vi "Lab Panel V5.25.1.vi"() -> ()   [LabVIEW 2013] (continued)
                            n2538 = local write "data file error"(w4596) -> ()
                          }
                        }
                      }
                    }
                  }
                }
              }
              frame #8 {
                n2539 = case shown="True" w4635 {
                  tunnel: w4639 -> [_ w4644]
                  tunnel: w4638 -> [_ w4643]
                  tunnel: w4637 -> [_ w4641]
                  tunnel: w4636 -> [_ w4640]
                  frame False {
                  }
                  frame True {
                    n2540 = local read "DISP LAB05-1"() -> (w4645:T4)
                    n2541 = local read "SIG LAB05-1"() -> (w4646:T2)
                    n2542 = local read "ON L05-1"() -> (w4642:cluster{"amps":dbl, "volts":dbl, "pf":dbl})
                    n2543 = Unbundle(w4646) -> ("AMPS"=w4652:dbl, "VOLTS"=w4650:dbl, "PF"=w4649:dbl, "Tmp Live"=w4648:dbl, "Tmp Neut"=w4651:dbl)
                    n2544 = Unbundle(w4645) -> ("CYCLE"=w4647:dbl)  [unwired: 2 out]
                    n2545 = stacked-sequence {
                      tunnel: w4652 -> [w4656 w4675]
                      tunnel: w4651 -> [_ w4674]
                      tunnel: w4650 -> [w4655 w4673]
                      tunnel: w4649 -> [w4654 w4672]
                      tunnel: w4648 -> [_ w4671]
                      tunnel: w4647 -> [_ w4670]
                      tunnel: w4644 -> [_ w4669]
                      tunnel: w4643 -> [w4657 _]
                      tunnel: w4642 -> [w4653 w4667]
                      tunnel: w4641 -> [_ w4668]
                      tunnel: w4640 -> [_ w4663]
                      frame #0 {
                        n2546 = case shown="True" w4657 {
                          tunnel: w4656 -> [_ w4662]
                          tunnel: w4655 -> [_ w4661]
                          tunnel: w4654 -> [_ w4660]
                          tunnel: w4653 -> [_ w4658]
                          frame False {
                          }
                          frame True {
                            n2547 = Bundle(cluster=w4658, "amps"=w4662, "volts"=w4661, "pf"=w4660) -> (w4659:cluster{"amps":dbl, "volts":dbl, "pf":dbl})
                            n2548 = local write "ON L05-1"(w4659) -> ()
                          }
                        }
                      }
                      frame #1 {
                        n2549 = Unbundle(w4667) -> ("amps"=w4666:dbl, "volts"=w4665:dbl, "pf"=w4664:dbl)
                        n2550 = case shown="True" w4668 {
                          tunnel: w4675 -> [_ w4707]
                          tunnel: w4674 -> [_ w4714]
                          tunnel: w4673 -> [_ _]
                          tunnel: w4672 -> [_ _]
                          tunnel: w4671 -> [_ w4713]
                          tunnel: w4670 -> [_ w4712]
                          tunnel: w4669 -> [_ w4677]
                          tunnel: w4666 -> [_ w4709]
                          tunnel: w4665 -> [_ w4708]
                          tunnel: w4664 -> [_ w4706]
                          tunnel: w4663 -> [_ w4698]
                          frame False {
                          }
                          frame True {
                            n2551 = local read "TDMS LAB05-1"() -> (w4711:refnum<k34>)
                            n2552 = Build Array(w4708) -> (w4703:dbl[])
                            n2553 = Build Array(w4706) -> (w4702:dbl[])
                            n2554 = Build Array(w4713) -> (w4701:dbl[])
                            n2555 = Build Array(w4714) -> (w4700:dbl[])
                            n2556 = Build Array(w4709) -> (w4705:dbl[])
                            n2557 = Build Array(w4707) -> (w4704:dbl[])
                            n2558 = Build Array(w4712) -> (w4699:dbl[])
                            n2559 = Build Array("AMPS ON", "AMPS OFF", "VOLTS", "PF", "TEMP Live", "TEMP Neut", "CYCLE") -> (w4682:string[])
                            n2560 = Bundle By Name("Y"=w4705, "t0"=w4698) -> (w4697:waveform(dbl))  [unwired: 1 in]
                            n2561 = Bundle By Name("Y"=w4704, "t0"=w4698) -> (w4696:waveform(dbl))  [unwired: 1 in]
                            n2562 = Bundle By Name("Y"=w4703, "t0"=w4698) -> (w4695:waveform(dbl))  [unwired: 1 in]
                            n2563 = Bundle By Name("Y"=w4702, "t0"=w4698) -> (w4694:waveform(dbl))  [unwired: 1 in]
                            n2564 = Bundle By Name("Y"=w4701, "t0"=w4698) -> (w4693:waveform(dbl))  [unwired: 1 in]
                            n2565 = Bundle By Name("Y"=w4700, "t0"=w4698) -> (w4692:waveform(dbl))  [unwired: 1 in]
                            n2566 = Bundle By Name("Y"=w4699, "t0"=w4698) -> (w4691:waveform(dbl))  [unwired: 1 in]
                            n2567 = Build Array(w4697, w4696, w4695, w4694, w4693, w4692, w4691) -> (w4690:waveform(dbl)[])
                            n2568 = TDMS Write(0:w4711, 5:"TEST VALUES", 7:w4682, 9:w4690) -> (4:w4681:refnum<k34>, 6:w4680:string, 15:w4679:errorcluster)  [unwired: 2 in, 1 out]
                            n2569 = TDMS Write(0:w4681, 5:w4680, 7:"TIME", 9:w4677, 11:w4679) -> (15:w4676:errorcluster)  [unwired: 1 in, 3 out]
                            n2570 = local write "data file error"(w4676) -> ()
                          }
                        }
                      }
                    }
                  }
                }
              }
              frame #9 {
                n2571 = case shown="True" w4715 {
                  tunnel: w4719 -> [_ w4724]
                  tunnel: w4718 -> [_ w4723]
                  tunnel: w4717 -> [_ w4721]
                  tunnel: w4716 -> [_ w4720]
                  frame False {
                  }
                  frame True {
                    n2572 = local read "DISP LAB05-2"() -> (w4725:T4)
                    n2573 = local read "SIG LAB05-2"() -> (w4726:T2)
                    n2574 = local read "ON L05-2"() -> (w4722:cluster{"amps":dbl, "volts":dbl, "pf":dbl})
                    n2575 = Unbundle(w4726) -> ("AMPS"=w4732:dbl, "VOLTS"=w4730:dbl, "PF"=w4729:dbl, "Tmp Live"=w4728:dbl, "Tmp Neut"=w4731:dbl)
                    n2576 = Unbundle(w4725) -> ("CYCLE"=w4727:dbl)  [unwired: 2 out]
                    n2577 = stacked-sequence {
                      tunnel: w4732 -> [w4736 w4755]
                      tunnel: w4731 -> [_ w4754]
                      tunnel: w4730 -> [w4735 w4753]
                      tunnel: w4729 -> [w4734 w4752]
                      tunnel: w4728 -> [_ w4751]
                      tunnel: w4727 -> [_ w4750]
                      tunnel: w4724 -> [_ w4749]
                      tunnel: w4723 -> [w4737 _]
                      tunnel: w4722 -> [w4733 w4747]
                      tunnel: w4721 -> [_ w4748]
                      tunnel: w4720 -> [_ w4743]
                      frame #0 {
                        n2578 = case shown="True" w4737 {
                          tunnel: w4736 -> [_ w4742]
                          tunnel: w4735 -> [_ w4741]
                          tunnel: w4734 -> [_ w4740]
                          tunnel: w4733 -> [_ w4738]
                          frame False {
                          }
                          frame True {
                            n2579 = Bundle(cluster=w4738, "amps"=w4742, "volts"=w4741, "pf"=w4740) -> (w4739:cluster{"amps":dbl, "volts":dbl, "pf":dbl})
                            n2580 = local write "ON L05-2"(w4739) -> ()
                          }
                        }
                      }
                      frame #1 {
                        n2581 = Unbundle(w4747) -> ("amps"=w4746:dbl, "volts"=w4745:dbl, "pf"=w4744:dbl)
                        n2582 = case shown="True" w4748 {
                          tunnel: w4755 -> [_ w4787]
                          tunnel: w4754 -> [_ w4794]
                          tunnel: w4753 -> [_ _]
                          tunnel: w4752 -> [_ _]
                          tunnel: w4751 -> [_ w4793]
                          tunnel: w4750 -> [_ w4792]
                          tunnel: w4749 -> [_ w4757]
                          tunnel: w4746 -> [_ w4789]
                          tunnel: w4745 -> [_ w4788]
                          tunnel: w4744 -> [_ w4786]
                          tunnel: w4743 -> [_ w4778]
                          frame False {
                          }
                          frame True {
                            n2583 = local read "TDMS LAB05-2"() -> (w4791:refnum<k34>)
                            n2584 = Build Array(w4788) -> (w4783:dbl[])
                            n2585 = Build Array(w4786) -> (w4782:dbl[])
                            n2586 = Build Array(w4793) -> (w4781:dbl[])
                            n2587 = Build Array(w4794) -> (w4780:dbl[])
                            n2588 = Build Array(w4789) -> (w4785:dbl[])
                            n2589 = Build Array(w4787) -> (w4784:dbl[])
                            n2590 = Build Array(w4792) -> (w4779:dbl[])
                            n2591 = Build Array("AMPS ON", "AMPS OFF", "VOLTS", "PF", "TEMP Live", "TEMP Neut", "CYCLE") -> (w4762:string[])
                            n2592 = Bundle By Name("Y"=w4785, "t0"=w4778) -> (w4777:waveform(dbl))  [unwired: 1 in]
                            n2593 = Bundle By Name("Y"=w4784, "t0"=w4778) -> (w4776:waveform(dbl))  [unwired: 1 in]
                            n2594 = Bundle By Name("Y"=w4783, "t0"=w4778) -> (w4775:waveform(dbl))  [unwired: 1 in]
                            n2595 = Bundle By Name("Y"=w4782, "t0"=w4778) -> (w4774:waveform(dbl))  [unwired: 1 in]
                            n2596 = Bundle By Name("Y"=w4781, "t0"=w4778) -> (w4773:waveform(dbl))  [unwired: 1 in]
                            n2597 = Bundle By Name("Y"=w4780, "t0"=w4778) -> (w4772:waveform(dbl))  [unwired: 1 in]
                            n2598 = Bundle By Name("Y"=w4779, "t0"=w4778) -> (w4771:waveform(dbl))  [unwired: 1 in]
                            n2599 = Build Array(w4777, w4776, w4775, w4774, w4773, w4772, w4771) -> (w4770:waveform(dbl)[])
                            n2600 = TDMS Write(0:w4791, 5:"TEST VALUES", 7:w4762, 9:w4770) -> (4:w4761:refnum<k34>, 6:w4760:string, 15:w4759:errorcluster)  [unwired: 2 in, 1 out]
                            n2601 = TDMS Write(0:w4761, 5:w4760, 7:"TIME", 9:w4757, 11:w4759) -> (15:w4756:errorcluster)  [unwired: 1 in, 3 out]
                            n2602 = local write "data file error"(w4756) -> ()
                          }
                        }
                      }
                    }
                  }
                }
              }
            }
          }
          frame #15 {
            # "display test values on chart"
            n2603 = local read "jig cycle"() -> (w4799:dbl)
            n2604 = local read "on loops"() -> (w4801:dbl)
            n2605 = Add(x=w4801, y=4) -> (x+y=w4798:dbl)
            n2606 = Equal?(x=w4799, y=3) -> (x = y?=w4797:bool)
            n2607 = Equal?(x=w4799, y=w4798) -> (x = y?=w4796:bool)
            n2608 = Or(x=w4797, y=w4796) -> (x .or. y?=w4795:bool)
            "graph flag" <- w4795
            n2609 = global write "Global display 3.vi" "graph flag"(w4795) -> ()
            n2610 = case shown="True" w4795 {
              frame False {
              }
              frame True {
                n2611 = local read "SIG LAB05-1"() -> (w4844:T2)
                n2612 = local read "SIG LAB04-2"() -> (w4845:T2)
                n2613 = local read "SIG LAB05-2"() -> (w4843:T2)
                n2614 = local read "SIG LAB04-1"() -> (w4846:T2)
                n2615 = local read "SIG LAB03-1"() -> (w4848:T2)
                n2616 = local read "SIG LAB03-2"() -> (w4847:T2)
                n2617 = local read "SIG LAB01-1"() -> (w4852:T2)
                n2618 = local read "SIG LAB02-2"() -> (w4849:T2)
                n2619 = local read "SIG LAB02-1"() -> (w4850:T2)
                n2620 = local read "SIG LAB01-2"() -> (w4851:T2)
                n2621 = Unbundle(w4845) -> ("AMPS"=w4835:dbl, "VOLTS"=w4825:dbl, "Tmp Live"=w4815:dbl, "Tmp Neut"=w4805:dbl)  [unwired: 1 out]
                n2622 = Unbundle(w4844) -> ("AMPS"=w4834:dbl, "VOLTS"=w4824:dbl, "Tmp Live"=w4814:dbl, "Tmp Neut"=w4804:dbl)  [unwired: 1 out]
                n2623 = Unbundle(w4843) -> ("AMPS"=w4833:dbl, "VOLTS"=w4823:dbl, "Tmp Live"=w4813:dbl, "Tmp Neut"=w4803:dbl)  [unwired: 1 out]
                n2624 = Unbundle(w4846) -> ("AMPS"=w4836:dbl, "VOLTS"=w4826:dbl, "Tmp Live"=w4816:dbl, "Tmp Neut"=w4806:dbl)  [unwired: 1 out]
                n2625 = Unbundle(w4847) -> ("AMPS"=w4837:dbl, "VOLTS"=w4827:dbl, "Tmp Live"=w4817:dbl, "Tmp Neut"=w4807:dbl)  [unwired: 1 out]
                n2626 = Unbundle(w4848) -> ("AMPS"=w4838:dbl, "VOLTS"=w4828:dbl, "Tmp Live"=w4818:dbl, "Tmp Neut"=w4808:dbl)  [unwired: 1 out]
                n2627 = Unbundle(w4849) -> ("AMPS"=w4839:dbl, "VOLTS"=w4829:dbl, "Tmp Live"=w4819:dbl, "Tmp Neut"=w4809:dbl)  [unwired: 1 out]
                n2628 = Unbundle(w4850) -> ("AMPS"=w4840:dbl, "VOLTS"=w4830:dbl, "Tmp Live"=w4820:dbl, "Tmp Neut"=w4810:dbl)  [unwired: 1 out]
                n2629 = Unbundle(w4852) -> ("AMPS"=w4842:dbl, "VOLTS"=w4832:dbl, "Tmp Live"=w4822:dbl, "Tmp Neut"=w4812:dbl)  [unwired: 1 out]
                n2630 = Unbundle(w4851) -> ("AMPS"=w4841:dbl, "VOLTS"=w4831:dbl, "Tmp Live"=w4821:dbl, "Tmp Neut"=w4811:dbl)  [unwired: 1 out]
                n2631 = stacked-sequence {
                  tunnel: w4842 -> [w4884 _ _]
                  tunnel: w4841 -> [w4883 _ _]
                  tunnel: w4840 -> [w4874 _ _]
                  tunnel: w4839 -> [w4873 _ _]
                  tunnel: w4838 -> [w4863 _ _]
                  tunnel: w4837 -> [w4862 _ _]
                  tunnel: w4836 -> [_ w4907 _]
                  tunnel: w4835 -> [_ w4906 _]
                  tunnel: w4834 -> [_ w4896 _]
                  tunnel: w4833 -> [_ w4895 _]
                  tunnel: w4832 -> [w4881 _ _]
                  tunnel: w4831 -> [w4880 _ _]
                  tunnel: w4830 -> [w4871 _ _]
                  tunnel: w4829 -> [w4870 _ _]
                  tunnel: w4828 -> [w4861 _ _]
                  tunnel: w4827 -> [w4860 _ _]
                  tunnel: w4826 -> [_ w4905 _]
                  tunnel: w4825 -> [_ w4904 _]
                  tunnel: w4824 -> [_ w4894 _]
                  tunnel: w4823 -> [_ w4893 _]
                  tunnel: w4822 -> [w4878 _ _]
                  tunnel: w4821 -> [w4876 _ _]
                  tunnel: w4820 -> [w4867 _ _]
                  tunnel: w4819 -> [w4865 _ _]
                  tunnel: w4818 -> [w4859 _ _]
                  tunnel: w4817 -> [w4857 _ _]
                  tunnel: w4816 -> [_ w4903 _]
                  tunnel: w4815 -> [_ w4901 _]
                  tunnel: w4814 -> [_ w4892 _]
                  tunnel: w4813 -> [_ w4890 _]
                  tunnel: w4812 -> [w4877 _ _]
                  tunnel: w4811 -> [w4875 _ _]
                  tunnel: w4810 -> [w4866 _ _]
                  tunnel: w4809 -> [w4864 _ _]
                  tunnel: w4808 -> [w4858 _ _]
                  tunnel: w4807 -> [w4856 _ _]
                  tunnel: w4806 -> [_ w4902 _]
                  tunnel: w4805 -> [_ w4900 _]
                  tunnel: w4804 -> [_ w4891 _]
                  tunnel: w4803 -> [_ w4889 _]
                  frame #0 {
                    n2632 = Merge Signals(w4884, w4883) -> (→"LAB01 AMPS":dynamicdata)
                    n2633 = Merge Signals(w4881, w4880) -> (→"LAB01 VOLTS":dynamicdata)
                    n2634 = Merge Signals(w4861, w4860) -> (→"LAB03 VOLTS":dynamicdata)
                    n2635 = Merge Signals(w4878, w4877, w4876, w4875) -> (→"LAB01 deg C":dynamicdata)
                    n2636 = Merge Signals(w4874, w4873) -> (→"LAB02 AMPS":dynamicdata)
                    n2637 = Merge Signals(w4867, w4866, w4865, w4864) -> (→"LAB02 deg C":dynamicdata)
                    n2638 = Merge Signals(w4859, w4858, w4857, w4856) -> (→"LAB03 deg C":dynamicdata)
                    n2639 = Merge Signals(w4871, w4870) -> (→"LAB02 VOLTS":dynamicdata)
                    n2640 = Merge Signals(w4863, w4862) -> (→"LAB03 AMPS":dynamicdata)
                  }
                  frame #1 {
                    n2641 = Merge Signals(w4894, w4893) -> (→"LAB05 VOLTS":dynamicdata)
                    n2642 = Merge Signals(w4907, w4906) -> (→"LAB04 AMPS":dynamicdata)
                    n2643 = Merge Signals(w4896, w4895) -> (→"LAB05 AMPS":dynamicdata)
                    n2644 = Merge Signals(w4892, w4891, w4890, w4889) -> (→"LAB05 deg C":dynamicdata)
                    n2645 = Merge Signals(w4903, w4902, w4901, w4900) -> (→"LAB04 deg C":dynamicdata)
                    n2646 = Merge Signals(w4905, w4904) -> (→"LAB04 VOLTS":dynamicdata)
                  }
                  frame #2 {
                    n2647 = local read "LAB05 VOLTS"() -> (w4915:dynamicdata)
                    n2648 = local read "LAB04 VOLTS"() -> (w4916:dynamicdata)
                    n2649 = local read "LAB02 VOLTS"() -> (w4918:dynamicdata)
                    n2650 = local read "LAB03 VOLTS"() -> (w4917:dynamicdata)
                    n2651 = local read "LAB05 AMPS"() -> (w4921:dynamicdata)
                    n2652 = local read "LAB01 VOLTS"() -> (w4919:dynamicdata)
                    n2653 = local read "LAB04 AMPS"() -> (w4922:dynamicdata)
                    n2654 = local read "LAB03 AMPS"() -> (w4923:dynamicdata)
                    n2655 = local read "LAB03 deg C"() -> (w4911:dynamicdata)
                    n2656 = local read "LAB02 AMPS"() -> (w4924:dynamicdata)
                    n2657 = local read "LAB04 deg C"() -> (w4910:dynamicdata)
                    n2658 = local read "LAB05 deg C"() -> (w4909:dynamicdata)
                    n2659 = local read "LAB02 deg C"() -> (w4912:dynamicdata)
                    n2660 = local read "LAB01 deg C"() -> (w4913:dynamicdata)
                    n2661 = local read "LAB01 AMPS"() -> (w4925:dynamicdata)
                    n2662 = Merge Signals(w4913, w4912, w4911, w4910, w4909) -> (w4908:dynamicdata)
                    n2663 = Merge Signals(w4925, w4924, w4923, w4922, w4921) -> (w4920:dynamicdata)
                    n2664 = Merge Signals(w4919, w4918, w4917, w4916, w4915) -> (w4914:dynamicdata)
                    n2665 = global write "Global display 3.vi" "graph volts"(w4914) -> ()
                    n2666 = global write "Global display 3.vi" "graph deg C"(w4908) -> ()
                    n2667 = global write "Global display 3.vi" "graph amps"(w4920) -> ()
                  }
                }
              }
            }
          }
          frame #16 {
            # "check for amps fail"
            # "check for cycle test & temperature rise fail conditions"
            n2668 = local read "on loops"() -> (w4952:dbl)
            n2669 = local read "jig cycle"() -> (w4949:dbl)
            n2670 = local read "jig cycle"() -> (w4954:dbl)
            n2671 = Add(x=w4952, y=5.0) -> (x+y=w4950:dbl)
            n2672 = Equal?(x=w4949, y=w4950) -> (x = y?=w4945:bool)
            n2673 = local read "Fail Loops"() -> (w4926:dbl)
            n2674 = Equal?(x=w4954, y=3.0) -> (x = y?=w4947:bool)
            n2675 = global write "Global 1.vi" "fail count"(w4926) -> ()
            n2676 = stacked-sequence {
              tunnel: w4948 -> [w4957 _ _ _ _ _ _ _ _ _]
              tunnel: w4947 -> [w4958 w4978 w4998 w5018 w5038 w5058 w5078 w5098 w5118 w5138]
              tunnel: w4946 -> [w4955 _ _ _ _ _ _ _ _ _]
              tunnel: w4945 -> [w4956 w4977 w4997 w5017 w5037 w5057 w5077 w5097 w5117 w5137]
              tunnel: w4944 -> [_ w4976 _ _ _ _ _ _ _ _]
              tunnel: w4943 -> [_ w4975 _ _ _ _ _ _ _ _]
              tunnel: w4942 -> [_ _ w4996 _ _ _ _ _ _ _]
              tunnel: w4941 -> [_ _ w4995 _ _ _ _ _ _ _]
              tunnel: w4940 -> [_ _ _ w5016 _ _ _ _ _ _]
              tunnel: w4939 -> [_ _ _ w5015 _ _ _ _ _ _]
              tunnel: w4938 -> [_ _ _ _ w5036 _ _ _ _ _]
              tunnel: w4937 -> [_ _ _ _ w5035 _ _ _ _ _]
              tunnel: w4936 -> [_ _ _ _ _ w5056 _ _ _ _]
              tunnel: w4935 -> [_ _ _ _ _ w5055 _ _ _ _]
              tunnel: w4934 -> [_ _ _ _ _ _ w5076 _ _ _]
              tunnel: w4933 -> [_ _ _ _ _ _ w5075 _ _ _]
              tunnel: w4932 -> [_ _ _ _ _ _ _ w5096 _ _]
              tunnel: w4931 -> [_ _ _ _ _ _ _ w5095 _ _]
              tunnel: w4930 -> [_ _ _ _ _ _ _ _ w5116 _]
              tunnel: w4929 -> [_ _ _ _ _ _ _ _ w5115 _]
              tunnel: w4928 -> [_ _ _ _ _ _ _ _ _ w5136]
              tunnel: w4927 -> [_ _ _ _ _ _ _ _ _ w5135]
              frame #0 {
                # "LAB01-1"
                n2677 = case shown="True" w4955 {
                  tunnel: w4958 -> [_ w4971]
                  tunnel: w4957 -> [_ w4968]
                  tunnel: w4956 -> [_ w4967]
                  frame False {
                  }
                  frame True {
                    n2678 = local read "TEMP START LAB01-1"() -> (w4973:cluster{"TL":dbl, "TN":dbl})
                    n2679 = local read "RESULT LAB01-1"() -> (w4962:bool)
                    n2680 = local read "FAIL LAB01-1"() -> (w4965:cluster{"LO":dbl, "HI":dbl})
                    n2681 = local read "TDMS LAB01-1"() -> (w4972:refnum<k34>)
                    n2682 = local read "SET LAB01-1"() -> (w4969:T5)
                    n2683 = local read "DISP LAB01-1"() -> (w4970:T4)
                    n2684 = local read "SIG LAB01-1"() -> (w4974:T2)
                    n2685 = Bundle("FAIL LAB01-1"=w4965, "SIG LAB01-1"=w4974, "TEMP START LAB01-1"=w4973, "DISP LAB01-1"=w4970, "SET LAB01-1"=w4969, "TDMS LAB01-1"=w4972) -> (w4959:T33)  [unwired: 1 in]
                    n2686 = call "sub vi - cycle&temp fail v7.vi"("Amps Lo?"=w4971, "Input Cluster"=w4959, "SELECT"=w4968, "Amps Hi?"=w4967, "Result In"=w4962) -> ("(FAIL) out"=w4964:cluster{"FAIL LO":dbl, "FAIL HI":dbl}, "(DISP) out"=w4960:T4, "T-RISE"=w4961:cluster{"T-RISE (L)":dbl, "T-RISE (N)":dbl}, "Result Out"=w4963:bool, "file error"=w4966:errorcluster)  [unwired: 10 in]
                    n2687 = local write "TEMP RISE LAB01-1"(w4961) -> ()
                    n2688 = local write "FAIL LAB01-1"(w4964) -> ()
                    n2689 = local write "DISP LAB01-1"(w4960) -> ()
                    n2690 = local write "RESULT LAB01-1"(w4963) -> ()
                    n2691 = local write "data file error"(w4966) -> ()
                  }
                }
              }
              frame #1 {
                # "LAB01-2"
                n2692 = case shown="True" w4976 {
                  tunnel: w4978 -> [_ w4991]
                  tunnel: w4975 -> [_ w4988]
                  tunnel: w4977 -> [_ w4987]
                  frame False {
                  }
                  frame True {
                    n2693 = local read "TEMP START LAB01-2"() -> (w4993:cluster{"TL":dbl, "TN":dbl})
                    n2694 = local read "FAIL LAB01-2"() -> (w4984:cluster{"LO":dbl, "HI":dbl})
                    n2695 = local read "TDMS LAB01-2"() -> (w4992:refnum<k34>)
                    n2696 = local read "SET LAB01-2"() -> (w4989:T5)
                    n2697 = local read "DISP LAB01-2"() -> (w4990:T4)
                    n2698 = local read "RESULT LAB01-2"() -> (w4981:bool)
                    n2699 = local read "SIG LAB01-2"() -> (w4994:T2)
                    n2700 = Bundle("FAIL LAB01-2"=w4984, "SIG LAB01-2"=w4994, "TEMP START LAB01-2"=w4993, "DISP LAB01-2"=w4990, "SET LAB01-2"=w4989, "TDMS LAB01-2"=w4992) -> (w4979:T34)  [unwired: 1 in]
                    n2701 = call "sub vi - cycle&temp fail v7.vi"("Amps Lo?"=w4991, "Input Cluster"=w4979, "SELECT"=w4988, "Amps Hi?"=w4987, "Result In"=w4981) -> ("(FAIL) out"=w4983:cluster{"FAIL LO":dbl, "FAIL HI":dbl}, "(DISP) out"=w4986:T4, "T-RISE"=w4980:cluster{"T-RISE (L)":dbl, "T-RISE (N)":dbl}, "Result Out"=w4982:bool, "file error"=w4985:errorcluster)  [unwired: 10 in]
                    n2702 = local write "TEMP RISE LAB01-2"(w4980) -> ()
                    n2703 = local write "FAIL LAB01-2"(w4983) -> ()
                    n2704 = local write "DISP LAB01-2"(w4986) -> ()
                    n2705 = local write "RESULT LAB01-2"(w4982) -> ()
                    n2706 = local write "data file error"(w4985) -> ()
                  }
                }
              }
              frame #2 {
                # "LAB02-1"
                n2707 = case shown="True" w4996 {
                  tunnel: w4998 -> [_ w5011]
                  tunnel: w4995 -> [_ w5008]
                  tunnel: w4997 -> [_ w5007]
                  frame False {
                  }
                  frame True {
                    n2708 = local read "TEMP START LAB02-1"() -> (w5013:cluster{"TL":dbl, "TN":dbl})
                    n2709 = local read "FAIL LAB02-1"() -> (w5004:cluster{"LO":dbl, "HI":dbl})
                    n2710 = local read "TDMS LAB02-1"() -> (w5012:refnum<k34>)
                    n2711 = local read "SET LAB02-1"() -> (w5009:T5)
                    n2712 = local read "DISP LAB02-1"() -> (w5010:T4)
                    n2713 = local read "SIG LAB02-1"() -> (w5014:T2)
                    n2714 = local read "RESULT LAB02-1"() -> (w5001:bool)
                    n2715 = Bundle("FAIL LAB02-1"=w5004, "SIG LAB02-1"=w5014, "TEMP START LAB02-1"=w5013, "DISP LAB02-1"=w5010, "SET LAB02-1"=w5009, "TDMS LAB02-1"=w5012) -> (w4999:T35)  [unwired: 1 in]
                    n2716 = call "sub vi - cycle&temp fail v7.vi"("Amps Lo?"=w5011, "Input Cluster"=w4999, "SELECT"=w5008, "Amps Hi?"=w5007, "Result In"=w5001) -> ("(FAIL) out"=w5003:cluster{"FAIL LO":dbl, "FAIL HI":dbl}, "(DISP) out"=w5006:T4, "T-RISE"=w5000:cluster{"T-RISE (L)":dbl, "T-RISE (N)":dbl}, "Result Out"=w5002:bool, "file error"=w5005:errorcluster)  [unwired: 10 in]
                    n2717 = local write "TEMP RISE LAB02-1"(w5000) -> ()
                    n2718 = local write "FAIL LAB02-1"(w5003) -> ()
                    n2719 = local write "DISP LAB02-1"(w5006) -> ()
                    n2720 = local write "RESULT LAB02-1"(w5002) -> ()
                    n2721 = local write "data file error"(w5005) -> ()
                  }
                }
              }
              frame #3 {
                # "LAB02-2"
                n2722 = case shown="True" w5016 {
                  tunnel: w5018 -> [_ w5031]
                  tunnel: w5015 -> [_ w5028]
                  tunnel: w5017 -> [_ w5027]
                  frame False {
                  }
                  frame True {
                    n2723 = local read "TEMP START LAB02-2"() -> (w5033:cluster{"TL":dbl, "TN":dbl})
                    n2724 = local read "FAIL LAB02-2"() -> (w5024:cluster{"LO":dbl, "HI":dbl})
                    n2725 = local read "TDMS LAB02-2"() -> (w5032:refnum<k34>)
                    n2726 = local read "SET LAB02-2"() -> (w5029:T5)
                    n2727 = local read "DISP LAB02-2"() -> (w5030:T4)
                    n2728 = local read "SIG LAB02-2"() -> (w5034:T2)
                    n2729 = local read "RESULT LAB02-2"() -> (w5021:bool)
                    n2730 = Bundle("FAIL LAB02-2"=w5024, "SIG LAB02-2"=w5034, "TEMP START LAB02-2"=w5033, "DISP LAB02-2"=w5030, "SET LAB02-2"=w5029, "TDMS LAB02-2"=w5032) -> (w5019:T36)  [unwired: 1 in]
                    n2731 = call "sub vi - cycle&temp fail v7.vi"("Amps Lo?"=w5031, "Input Cluster"=w5019, "SELECT"=w5028, "Amps Hi?"=w5027, "Result In"=w5021) -> ("(FAIL) out"=w5023:cluster{"FAIL LO":dbl, "FAIL HI":dbl}, "(DISP) out"=w5026:T4, "T-RISE"=w5020:cluster{"T-RISE (L)":dbl, "T-RISE (N)":dbl}, "Result Out"=w5022:bool, "file error"=w5025:errorcluster)  [unwired: 10 in]
                    n2732 = local write "TEMP RISE LAB02-2"(w5020) -> ()
                    n2733 = local write "FAIL LAB02-2"(w5023) -> ()
                    n2734 = local write "DISP LAB02-2"(w5026) -> ()
                    n2735 = local write "RESULT LAB02-2"(w5022) -> ()
                    n2736 = local write "data file error"(w5025) -> ()
                  }
                }
              }
              frame #4 {
                # "LAB03-1"
                n2737 = case shown="True" w5036 {
                  tunnel: w5038 -> [_ w5051]
                  tunnel: w5035 -> [_ w5048]
                  tunnel: w5037 -> [_ w5047]
                  frame False {
                  }
                  frame True {
                    n2738 = local read "TEMP START LAB03-1"() -> (w5053:cluster{"TL":dbl, "TN":dbl})
                    n2739 = local read "FAIL LAB03-1"() -> (w5044:cluster{"LO":dbl, "HI":dbl})
                    n2740 = local read "TDMS LAB03-1"() -> (w5052:refnum<k34>)
                    n2741 = local read "SET LAB03-1"() -> (w5049:T5)
                    n2742 = local read "DISP LAB03-1"() -> (w5050:T4)
                    n2743 = local read "SIG LAB03-1"() -> (w5054:T2)
                    n2744 = local read "RESULT LAB03-1"() -> (w5041:bool)
                    n2745 = Bundle("FAIL LAB03-1"=w5044, "SIG LAB03-1"=w5054, "TEMP START LAB03-1"=w5053, "DISP LAB03-1"=w5050, "SET LAB03-1"=w5049, "TDMS LAB03-1"=w5052) -> (w5039:T37)  [unwired: 1 in]
                    n2746 = call "sub vi - cycle&temp fail v7.vi"("Amps Lo?"=w5051, "Input Cluster"=w5039, "SELECT"=w5048, "Amps Hi?"=w5047, "Result In"=w5041) -> ("(FAIL) out"=w5043:cluster{"FAIL LO":dbl, "FAIL HI":dbl}, "(DISP) out"=w5046:T4, "T-RISE"=w5040:cluster{"T-RISE (L)":dbl, "T-RISE (N)":dbl}, "Result Out"=w5042:bool, "file error"=w5045:errorcluster)  [unwired: 10 in]
                    n2747 = local write "TEMP RISE LAB03-1"(w5040) -> ()
                    n2748 = local write "FAIL LAB03-1"(w5043) -> ()
                    n2749 = local write "DISP LAB03-1"(w5046) -> ()
                    n2750 = local write "RESULT LAB03-1"(w5042) -> ()
                    n2751 = local write "data file error"(w5045) -> ()
                  }
                }
              }
              frame #5 {
                # "LAB03-2"
                n2752 = case shown="True" w5056 {
                  tunnel: w5058 -> [_ w5071]
                  tunnel: w5055 -> [_ w5068]
                  tunnel: w5057 -> [_ w5067]
                  frame False {
                  }
                  frame True {
                    n2753 = local read "TEMP START LAB03-2"() -> (w5073:cluster{"TL":dbl, "TN":dbl})
                    n2754 = local read "FAIL LAB03-2"() -> (w5064:cluster{"LO":dbl, "HI":dbl})
                    n2755 = local read "TDMS LAB03-2"() -> (w5072:refnum<k34>)
                    n2756 = local read "SET LAB03-2"() -> (w5069:T5)
                    n2757 = local read "DISP LAB03-2"() -> (w5070:T4)
                    n2758 = local read "RESULT LAB03-2"() -> (w5061:bool)
                    n2759 = local read "SIG LAB03-2"() -> (w5074:T2)
                    n2760 = Bundle("FAIL LAB03-2"=w5064, "SIG LAB03-2"=w5074, "TEMP START LAB03-2"=w5073, "DISP LAB03-2"=w5070, "SET LAB03-2"=w5069, "TDMS LAB03-2"=w5072) -> (w5059:T38)  [unwired: 1 in]
                    n2761 = call "sub vi - cycle&temp fail v7.vi"("Amps Lo?"=w5071, "Input Cluster"=w5059, "SELECT"=w5068, "Amps Hi?"=w5067, "Result In"=w5061) -> ("(FAIL) out"=w5063:cluster{"FAIL LO":dbl, "FAIL HI":dbl}, "(DISP) out"=w5066:T4, "T-RISE"=w5060:cluster{"T-RISE (L)":dbl, "T-RISE (N)":dbl}, "Result Out"=w5062:bool, "file error"=w5065:errorcluster)  [unwired: 10 in]
                    n2762 = local write "FAIL LAB03-2"(w5063) -> ()
                    n2763 = local write "TEMP RISE LAB03-2"(w5060) -> ()
                    n2764 = local write "DISP LAB03-2"(w5066) -> ()
                    n2765 = local write "RESULT LAB03-2"(w5062) -> ()
                    n2766 = local write "data file error"(w5065) -> ()
                  }
                }
              }
              frame #6 {
                # "LAB04-1"
                n2767 = case shown="True" w5076 {
                  tunnel: w5078 -> [_ w5091]
                  tunnel: w5075 -> [_ w5088]
                  tunnel: w5077 -> [_ w5087]
                  frame False {
                  }
                  frame True {
                    n2768 = local read "TEMP START LAB04-1"() -> (w5093:cluster{"TL":dbl, "TN":dbl})
                    n2769 = local read "FAIL LAB04-1"() -> (w5084:cluster{"LO":dbl, "HI":dbl})
                    n2770 = local read "TDMS LAB04-1"() -> (w5092:refnum<k34>)
                    n2771 = local read "SET LAB04-1"() -> (w5089:T5)
                    n2772 = local read "DISP LAB04-1"() -> (w5090:T4)
                    n2773 = local read "SIG LAB04-1"() -> (w5094:T2)
                    n2774 = local read "RESULT LAB04-1"() -> (w5081:bool)
                    n2775 = Bundle("FAIL LAB04-1"=w5084, "SIG LAB04-1"=w5094, "TEMP START LAB04-1"=w5093, "DISP LAB04-1"=w5090, "SET LAB04-1"=w5089, "TDMS LAB04-1"=w5092) -> (w5079:T39)  [unwired: 1 in]
                    n2776 = call "sub vi - cycle&temp fail v7.vi"("Amps Lo?"=w5091, "Input Cluster"=w5079, "SELECT"=w5088, "Amps Hi?"=w5087, "Result In"=w5081) -> ("(FAIL) out"=w5083:cluster{"FAIL LO":dbl, "FAIL HI":dbl}, "(DISP) out"=w5086:T4, "T-RISE"=w5080:cluster{"T-RISE (L)":dbl, "T-RISE (N)":dbl}, "Result Out"=w5082:bool, "file error"=w5085:errorcluster)  [unwired: 10 in]
                    n2777 = local write "TEMP RISE LAB04-1"(w5080) -> ()
                    n2778 = local write "FAIL LAB04-1"(w5083) -> ()
                    n2779 = local write "DISP LAB04-1"(w5086) -> ()
                    n2780 = local write "RESULT LAB04-1"(w5082) -> ()
                    n2781 = local write "data file error"(w5085) -> ()
                  }
                }
              }
              frame #7 {
                # "LAB04-2"
                n2782 = case shown="True" w5096 {
                  tunnel: w5098 -> [_ w5111]
                  tunnel: w5095 -> [_ w5108]
                  tunnel: w5097 -> [_ w5107]
                  frame False {
                  }
                  frame True {
                    n2783 = local read "TEMP START LAB04-2"() -> (w5113:cluster{"TL":dbl, "TN":dbl})
                    n2784 = local read "FAIL LAB04-2"() -> (w5104:cluster{"LO":dbl, "HI":dbl})
                    n2785 = local read "TDMS LAB04-2"() -> (w5112:refnum<k34>)
                    n2786 = local read "SET LAB04-2"() -> (w5109:T5)
                    n2787 = local read "DISP LAB04-2"() -> (w5110:T4)
                    n2788 = local read "SIG LAB04-2"() -> (w5114:T2)
                    n2789 = local read "RESULT LAB04-2"() -> (w5101:bool)
                    n2790 = Bundle("FAIL LAB04-2"=w5104, "SIG LAB04-2"=w5114, "TEMP START LAB04-2"=w5113, "DISP LAB04-2"=w5110, "SET LAB04-2"=w5109, "TDMS LAB04-2"=w5112) -> (w5099:T40)  [unwired: 1 in]
                    n2791 = call "sub vi - cycle&temp fail v7.vi"("Amps Lo?"=w5111, "Input Cluster"=w5099, "SELECT"=w5108, "Amps Hi?"=w5107, "Result In"=w5101) -> ("(FAIL) out"=w5103:cluster{"FAIL LO":dbl, "FAIL HI":dbl}, "(DISP) out"=w5106:T4, "T-RISE"=w5100:cluster{"T-RISE (L)":dbl, "T-RISE (N)":dbl}, "Result Out"=w5102:bool, "file error"=w5105:errorcluster)  [unwired: 10 in]
                    n2792 = local write "TEMP RISE LAB04-2"(w5100) -> ()
                    n2793 = local write "FAIL LAB04-2"(w5103) -> ()
                    n2794 = local write "DISP LAB04-2"(w5106) -> ()
                    n2795 = local write "RESULT LAB04-2"(w5102) -> ()
                    n2796 = local write "data file error"(w5105) -> ()
                  }
                }
              }
              frame #8 {
                # "LAB05-1"
                n2797 = case shown="True" w5116 {
                  tunnel: w5118 -> [_ w5131]
                  tunnel: w5115 -> [_ w5128]
                  tunnel: w5117 -> [_ w5127]
                  frame False {
                  }
                  frame True {
                    n2798 = local read "TEMP START LAB05-1"() -> (w5133:cluster{"TL":dbl, "TN":dbl})
                    n2799 = local read "FAIL LAB05-1"() -> (w5124:cluster{"LO":dbl, "HI":dbl})
                    n2800 = local read "TDMS LAB05-1"() -> (w5132:refnum<k34>)
                    n2801 = local read "SET LAB05-1"() -> (w5129:T5)
                    n2802 = local read "DISP LAB05-1"() -> (w5130:T4)
                    n2803 = local read "SIG LAB05-1"() -> (w5134:T2)
                    n2804 = local read "RESULT LAB05-1"() -> (w5121:bool)
                    n2805 = Bundle("FAIL LAB05-1"=w5124, "SIG LAB05-1"=w5134, "TEMP START LAB05-1"=w5133, "DISP LAB05-1"=w5130, "SET LAB05-1"=w5129, "TDMS LAB05-1"=w5132) -> (w5119:T41)  [unwired: 1 in]
                    n2806 = call "sub vi - cycle&temp fail v7.vi"("Amps Lo?"=w5131, "Input Cluster"=w5119, "SELECT"=w5128, "Amps Hi?"=w5127, "Result In"=w5121) -> ("(FAIL) out"=w5123:cluster{"FAIL LO":dbl, "FAIL HI":dbl}, "(DISP) out"=w5126:T4, "T-RISE"=w5120:cluster{"T-RISE (L)":dbl, "T-RISE (N)":dbl}, "Result Out"=w5122:bool, "file error"=w5125:errorcluster)  [unwired: 10 in]
                    n2807 = local write "TEMP RISE LAB05-1"(w5120) -> ()
                    n2808 = local write "FAIL LAB05-1"(w5123) -> ()
                    n2809 = local write "DISP LAB05-1"(w5126) -> ()
                    n2810 = local write "RESULT LAB05-1"(w5122) -> ()
                    n2811 = local write "data file error"(w5125) -> ()
                  }
                }
              }
              frame #9 {
                # "LAB05-2"
                n2812 = case shown="True" w5136 {
                  tunnel: w5138 -> [_ w5151]
                  tunnel: w5135 -> [_ w5148]
                  tunnel: w5137 -> [_ w5147]
                  frame False {
                  }
                  frame True {
                    n2813 = local read "TEMP START LAB05-2"() -> (w5153:cluster{"TL":dbl, "TN":dbl})
                    n2814 = local read "FAIL LAB05-2"() -> (w5144:cluster{"LO":dbl, "HI":dbl})
                    n2815 = local read "TDMS LAB05-2"() -> (w5152:refnum<k34>)
                    n2816 = local read "SET LAB05-2"() -> (w5149:T5)
                    n2817 = local read "DISP LAB05-2"() -> (w5150:T4)
                    n2818 = local read "SIG LAB05-2"() -> (w5154:T2)
                    n2819 = local read "RESULT LAB05-2"() -> (w5141:bool)
                    n2820 = Bundle("FAIL LAB05-2"=w5144, "SIG LAB05-2"=w5154, "TEMP START LAB05-2"=w5153, "DISP LAB05-2"=w5150, "SET LAB05-2"=w5149, "TDMS LAB05-2"=w5152) -> (w5139:T42)  [unwired: 1 in]
                    n2821 = call "sub vi - cycle&temp fail v7.vi"("Amps Lo?"=w5151, "Input Cluster"=w5139, "SELECT"=w5148, "Amps Hi?"=w5147, "Result In"=w5141) -> ("(FAIL) out"=w5143:cluster{"FAIL LO":dbl, "FAIL HI":dbl}, "(DISP) out"=w5146:T4, "T-RISE"=w5140:cluster{"T-RISE (L)":dbl, "T-RISE (N)":dbl}, "Result Out"=w5142:bool, "file error"=w5145:errorcluster)  [unwired: 10 in]
                    n2822 = local write "TEMP RISE LAB05-2"(w5140) -> ()
                    n2823 = local write "FAIL LAB05-2"(w5143) -> ()
                    n2824 = local write "DISP LAB05-2"(w5146) -> ()
                    n2825 = local write "RESULT LAB05-2"(w5142) -> ()
                    n2826 = local write "data file error"(w5145) -> ()
                  }
                }
              }
            }
          }
          frame #17 {
            # "run calibration routine"
            n2827 = local read "SET (cal)"() -> (w5155:bool)
            n2828 = case shown="True" w5155 {
              frame False {
              }
              frame True {
                n2829 = stacked-sequence {
                  seq-local: [w5156 _ _] -> [_ w5158 _]
                  frame #0 {
                    n2830 = call "CALIBRATION PASSWORD"() -> ("PASSWORD"=w5156:string)  [unwired: 17 in, 2 out]
                  }
                  frame #1 {
                    n2831 = Equal?(x=w5158, y="7777") -> (x = y?=w5157:bool)
                    n2832 = case shown="True" w5157 {
                      frame False {
                      }
                      frame True {
                        n2833 = stacked-sequence {
                          frame #0 {
                            n2834 = local read "Temp Test Cal"() -> (w5160:dbl)
                            n2835 = call "sub vi - calibration v1.vi"("Temp Test Cal"=w5160) -> ()  [unwired: 11 in]
                          }
                          frame #1 {
                            n2836 = call "sub vi - get calibration values v1.vi"() -> ("TEMP REF CAL"=w5161:dbl, "LAB01 (CAL)"=w5166:T14, "LAB02 (CAL)"=w5165:T15, "LAB03 (CAL)"=w5164:T14, "LAB04 (CAL)"=w5163:T14, "calibration file error out"=w5167:errorcluster, "LAB05 (CAL)"=w5162:T14)  [unwired: 9 in]
                            n2837 = local write "TEMP REF cal"(w5161) -> ()
                            n2838 = local write "cal file error out"(w5167) -> ()
                            n2839 = local write "CAL LAB04"(w5163) -> ()
                            n2840 = local write "CAL LAB05"(w5162) -> ()
                            n2841 = local write "CAL LAB01"(w5166) -> ()
                            n2842 = local write "CAL LAB02"(w5165) -> ()
                            n2843 = local write "CAL LAB03"(w5164) -> ()
                          }
                        }
                      }
                    }
                  }
                  frame #2 {
                    n2844 = local write "SET (cal)"(FALSE) -> ()
                  }
                }
              }
            }
          }
          frame #18 {
            # "save certain settings to file"
            n2845 = String To Path(string="c:\\crabtree\\Set Up\\") -> (path=w5170:path)
            n2846 = Build Path(base path=w5170, name or relative path="settings.bin") -> (appended path=w5172:path)
            n2847 = Build Path(base path=w5170, name or relative path="mail.bin") -> (appended path=w5169:path)
            n2848 = Create Folder(path (use dialog)=w5170) -> (error out=w5175:errorcluster)  [unwired: 2 in, 2 out]
            n2849 = call <vilib>:"Clear Errors.vi"("error in (no error)"=w5175) -> ()  [unwired: 6 in, 1 out]
            n2850 = stacked-sequence {
              seq-local: [w5188 _] -> [_ w5201]
              tunnel: w5172 -> [_ w5202]
              tunnel: w5169 -> [_ w5200]
              frame #0 {
                n2851 = local read "C drive data root dir"() -> (w5187:path)
                n2852 = local read "Select COM port"() -> (w5184:refnum<visa-resource-name>)
                n2853 = local read "Network Directory"() -> (w5193:path)
                n2854 = local read "SET LAB05-2"() -> (w5192:T5)
                n2855 = local read "SET LAB05-1"() -> (w5191:T5)
                n2856 = local read "SET LAB04-2"() -> (w5190:T5)
                n2857 = local read "SET LAB03-2"() -> (w5194:T5)
                n2858 = local read "SET LAB04-1"() -> (w5189:T5)
                n2859 = local read "SET LAB03-1"() -> (w5195:T5)
                n2860 = local read "SET LAB02-2"() -> (w5196:T5)
                n2861 = local read "SET LAB02-1"() -> (w5197:T5)
                n2862 = local read "Temp Delay Lps"() -> (w5183:dbl)
                n2863 = local read "Amps Fail level"() -> (w5179:dbl)
                n2864 = local read "SET LAB01-2"() -> (w5198:T5)
                n2865 = local read "Temp Test Cal"() -> (w5180:dbl)
                n2866 = local read "SET LAB01-1"() -> (w5199:T5)
                n2867 = local read "Mail Test File To:"() -> (w5178:string)
                n2868 = local read "Temp Value"() -> (w5182:dbl)
                n2869 = local read "Fail Loops"() -> (w5181:dbl)
                n2870 = local read "SAMPLES 2"() -> (w5176:dbl)
                n2871 = local read "Mail Test Fail"() -> (w5177:bool)
                n2872 = local read "RATE (Hz)"() -> (w5186:dbl)
                n2873 = local read "SAMPLES"() -> (w5185:dbl)
                n2874 = Bundle("SET LAB01-1"=w5199, "SET LAB01-2"=w5198, "SET LAB02-1"=w5197, "SET LAB02-2"=w5196, "SET LAB03-1"=w5195, "SET LAB03-2"=w5194, "SET LAB04-1"=w5189, "SET LAB04-2"=w5190, "SET LAB05-1"=w5191, "SET LAB05-2"=w5192, "Network Directory"=w5193, "C drive data root dir"=w5187, "RATE (Hz)"=w5186, "SAMPLES"=w5185, "Select COM port"=w5184, "Temp Delay Lps"=w5183, "Temp Value"=w5182, "Fail Loops"=w5181, "Temp Test Cal"=w5180, "Amps Fail level"=w5179, "Mail Test File To:"=w5178, "Mail Test Fail"=w5177, "SAMPLES 2"=w5176) -> (w5188:T22)  [unwired: 1 in]
              }
              frame #1 {
                n2875 = event shown="[1] \"SET LAB01-1\", \"SET LAB01-2\", \"SET LAB02-1\", \"SET LAB02-2\", \"SET LAB03-1\", \"SET LAB03-2\", \"SET LAB04-1\", \"SET LAB04-2\", \"SET LAB05-1\", \"SET LAB05-2\", \"Network Directory\", \"C drive data root dir\", \"RATE (Hz)\", \"SAMPLES\", \"Select COM port\", \"Temp Delay Lps\", \"Temp Value\", \"Fail Loops\", \"Temp Test Cal\", \"Amps Fail level\", \"Mail Test File To:\", \"Mail Test Fail\", \"SAMPLES 2\": Value Change" {
                  selector: _ -> [_ _ _]
                  dyn-events: _ -> [_ _ _]
                  timeout: 10.0 -> [_ _ _]
                  tunnel: w5202 -> [_ w5204 _]
                  tunnel: w5201 -> [_ w5205 _]
                  tunnel: w5200 -> [_ _ w5216]
                  event Timeout {
                    n2876 = event-data() -> ()  [unwired: 1 in, 3 out]
                  }
                  event "SET LAB01-1", "SET LAB01-2", "SET LAB02-1", "SET LAB02-2", "SET LAB03-1", "SET LAB03-2", "SET LAB04-1", "SET LAB04-2", "SET LAB05-1", "SET LAB05-2", "Network Directory", "C drive data root dir", "RATE (Hz)", "SAMPLES", "Select COM port", "Temp Delay Lps", "Temp Value", "Fail Loops", "Temp Test Cal", "Amps Fail level", "Mail Test File To:", "Mail Test Fail", "SAMPLES 2": Value Change {
                    n2877 = event-data() -> ()  [unwired: 1 in, 6 out]
                    n2878 = Open/Create/Replace File(file path (use dialog)=w5204, operation (0:open)=T17."replace or create") -> (refnum out=w5210:refnum<file>, error out=w5209:errorcluster)  [unwired: 4 in, 1 out]
                    n2879 = Write to Binary File(file (use dialog)=w5210, data=w5205, error in=w5209) -> (refnum out=w5208:refnum<file>, error out=w5207:errorcluster)  [unwired: 3 in, 1 out]
                    n2880 = Close File(refnum=w5208, error in=w5207) -> (error out=w5206:errorcluster)  [unwired: 1 out]
                    n2881 = local write "data file error"(w5206) -> ()
                  }
                  event "MAIL SETTINGS.OUT SERVER ADDRESS", "MAIL SETTINGS.FROM ACCOUNT", "MAIL SETTINGS.USER NAME", "MAIL SETTINGS.PASSWORD", "Auto Mail Send", "TO (string):": Value Change {
                    n2882 = event-data() -> ()  [unwired: 1 in, 6 out]
                    n2883 = local read "MAIL SETTINGS"() -> (w5215:T7)
                    n2884 = local read "Auto Mail Send"() -> (w5213:bool)
                    n2885 = local read "TO (string):"() -> (w5212:string)
                    n2886 = Open/Create/Replace File(file path (use dialog)=w5216, operation (0:open)=T17."replace or create") -> (refnum out=w5221:refnum<file>, error out=w5220:errorcluster)  [unwired: 4 in, 1 out]
                    n2887 = Bundle("MAIL SETTINGS"=w5215, "Auto Mail Send"=w5213, "TO (string):"=w5212) -> (w5214:T43)  [unwired: 1 in]
                    n2888 = Write to Binary File(file (use dialog)=w5221, data=w5214, error in=w5220) -> (refnum out=w5219:refnum<file>, error out=w5218:errorcluster)  [unwired: 3 in, 1 out]
                    n2889 = Close File(refnum=w5219, error in=w5218) -> (error out=w5217:errorcluster)  [unwired: 1 out]
                    n2890 = local write "data file error"(w5217) -> ()
                  }
                }
              }
            }
          }
          frame #19 {
            # "mail control"
            n2891 = local read "MAIL SETTINGS"() -> (w5238:T7)
            n2892 = local read "Auto Mail Send"() -> (w5224:bool)
            n2893 = Unbundle(w5238) -> ("OUT SERVER ADDRESS"=w5237:string, "FROM ACCOUNT"=w5236:string, "TEST MAIL"=w5235:bool)  [unwired: 4 out]
            n2894 = stacked-sequence {
              tunnel: "TO (string):" -> [_ w5277]
              tunnel: w5238 -> [w5243 w5276]
              tunnel: w5237 -> [w5242 w5275]
              tunnel: w5236 -> [w5241 w5274]
              tunnel: w5235 -> [w5240 _]
              tunnel: w5224 -> [_ w5273]
              tunnel: w5234 -> [_ w5272]
              tunnel: w5233 -> [_ w5271]
              tunnel: w5232 -> [_ w5270]
              tunnel: w5231 -> [_ w5269]
              tunnel: w5230 -> [_ w5268]
              tunnel: w5229 -> [_ w5267]
              tunnel: w5228 -> [_ w5266]
              tunnel: w5227 -> [_ w5265]
              tunnel: w5226 -> [_ w5264]
              tunnel: w5225 -> [_ w5263]
              tunnel: "TO (string):" -> [w5239 _]
              frame #0 {
                # "mail test"
                n2895 = case shown="True" w5240 {
                  tunnel: w5243 -> [_ w5247]
                  tunnel: w5239 -> [_ w5246]
                  tunnel: w5242 -> [_ w5245]
                  tunnel: w5241 -> [_ w5244]
                  frame False {
                  }
                  frame True {
                    n2896 = stacked-sequence {
                      seq-local: [_ _ w5257 _] -> [_ _ _ w5258]
                      tunnel: w5247 -> [w5250 _ _ w5262]
                      tunnel: w5246 -> [_ _ w5255 _]
                      tunnel: w5245 -> [_ _ w5253 _]
                      tunnel: w5244 -> [_ _ w5254 _]
                      frame #0 {
                        n2897 = Bundle(cluster=w5250, "TEST MAIL STATUS"="TEST START") -> (w5248:T7)  [unwired: 6 in]
                        n2898 = local write "MAIL SETTINGS"(w5248) -> ()
                      }
                      frame #1 {
                        n2899 = Wait (ms)(milliseconds to wait=500) -> ()  [unwired: 1 out]
                      }
                      frame #2 {
